vi "Actor Core.vi"(8 "error in":errorcluster, 11 "Panel Object Actions UI in":refnum<class "Panel Object Actions UI.lvclass">) -> (0 "error out":errorcluster, 3 "Actor out":refnum<class "Actor.lvclass">)   [LabVIEW 2019, in "Panel Object Actions UI.lvlib" / "Panel Object Actions UI.lvclass"]
doc: "The user interface for this panel.\n\n----\nPlease see the following web address for additional documentation and tutorial information:\nhttp://www.mooregoodideas.com/mgi-panel-manager/\n\nAuthor: Derek Trepanier\n\nCopyright (c) 2018, Moore Good Ideas, Inc.\n\nAll rights reserved.\n\nRedistribution and use in source and binary forms, with or without modification, are permitted provided that the following conditions are met:\n\n * Redistributions of source code must retain the above copyright notice, this list of conditions and the following disclaimer.\n * Redistributions in binary form must reproduce the above copyright notice, this list of conditions and the following disclaimer in the documentation and/or other materials provided with the distribution.\n * Neither the name of Moore Good Ideas, Inc. nor the names of its contributors may be used to endorse or promote products derived from this software without specific prior written permission.\n\nTHIS SOFTWARE IS PROVIDED BY THE COPYRIGHT HOLDERS AND CONTRIBUTORS \"AS IS\" AND ANY EXPRESS OR IMPLIED WARRANTIES, INCLUDING, BUT NOT LIMITED TO, THE IMPLIED WARRANTIES OF MERCHANTABILITY AND FITNESS FOR A PARTICULAR PURPOSE ARE DISCLAIMED. IN NO EVENT SHALL THE COPYRIGHT OWNER OR CONTRIBUTORS BE LIABLE FOR ANY DIRECT, INDIRECT, INCIDENTAL, SPECIAL, EXEMPLARY, OR CONSEQUENTIAL DAMAGES (INCLUDING, BUT NOT LIMITED TO, PROCUREMENT OF SUBSTITUTE GOODS OR SERVICES; LOSS OF USE, DATA, OR PROFITS; OR BUSINESS INTERRUPTION) HOWEVER CAUSED AND ON ANY THEORY OF LIABILITY, WHETHER IN CONTRACT, STRICT LIABILITY, OR TORT (INCLUDING NEGLIGENCE OR OTHERWISE) ARISING IN ANY WAY OUT OF THE USE OF THIS SOFTWARE, EVEN IF ADVISED OF THE POSSIBILITY OF SUCH DAMAGE."
uses:
  <resource>/dialog/QuickDrop/plugins/PaneRelief/Classes/Panel Object Actions UI/Panel Object Actions UI/Panel Object Actions UI.lvclass
  C:/Program Files (x86)/National Instruments/LabVIEW 2019/vi.lib/MGI/Panel Manager/Panel Actor/Panel Actor/Panel Actor.lvclass
  C:/Program Files (x86)/National Instruments/LabVIEW 2019/vi.lib/ActorFramework/Actor/Actor.lvclass
  <vilib>/ActorFramework/Actor/Actor.lvclass
  <resource>/dialog/QuickDrop/plugins/PaneRelief/Classes/Panel Object/Panel Object.lvclass
  <vilib>/ActorFramework/Actor/Actor.lvclass/Actor.ctl
  <resource>/dialog/QuickDrop/plugins/PaneRelief/Classes/Panel Object Actions UI/Panel Object Actions UI/Panel Object Actions UI.lvclass/Panel Object Actions UI.ctl
  <vilib>/ActorFramework/Message Enqueuer/Message Enqueuer.lvclass/Message Enqueuer.ctl
  <resource>/dialog/QuickDrop/plugins/PaneRelief/Typedefs/Scrollbar Visibility--Enum.ctl
  <resource>/dialog/QuickDrop/plugins/PaneRelief/Classes/Panel Object/Align Type--Enum.ctl
  <resource>/dialog/QuickDrop/plugins/PaneRelief/Classes/Panel Object/Distribution Type--Enum.ctl
  <vilib>/ActorFramework/Message Enqueuer/Enqueue.vi
  <resource>/dialog/QuickDrop/plugins/PaneRelief/Classes/Pane Relief Main UI/Pane Relief Main UI Messages/Panel Object Settings Changed Msg/Panel Object Settings Changed Msg.lvclass
  C:/Program Files (x86)/National Instruments/LabVIEW 2019/vi.lib/ActorFramework/Message/Message.lvclass
  <vilib>/ActorFramework/Message Priority Queue/Priority Enqueue.vi
  <vilib>/MGI/Panel Manager/Panel Actor/Panel Actor/Panel Actor.lvclass
  <vilib>/ActorFramework/Message Enqueuer/Message Enqueuer.lvclass
panel:
  in  "Scrollbars Off":bool
  in  "Scrollbars Off":bool
  in  "Unlock Splitters":bool
  in  "Lock Splitters":bool
  in  "Distribute Horizontally":bool
  in  "Distribute Vertically":bool
  in  "Set Color":bool
  in  "Scrollbars On":bool
  in  "Origin To (0,0)":bool
  in  "Align Right":bool
  in  "Align Bottom":bool
  in  "Align Left":bool
  in  "Align Top":bool
  in  "Color":u32(colorbox)
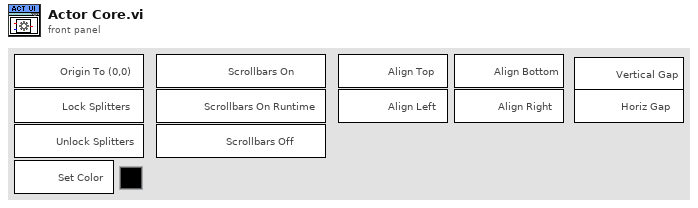
[diagram p1: front panel]
types:
  T1 = cluster{"Event Registration Refnum":refnum<event-registration>, "Pnl Actor":refnum<event-registration>}
  T2 = typedef "Scrollbar Visibility--Enum.ctl" = enum16{"On", "Off", "Off While Running"}
  T3 = typedef "Align Type--Enum.ctl" = enum16{"Top", "Bottom", "Left", "Right"}
  T4 = typedef "Distribution Type--Enum.ctl" = enum16{"Vertical", "Horizontal"}
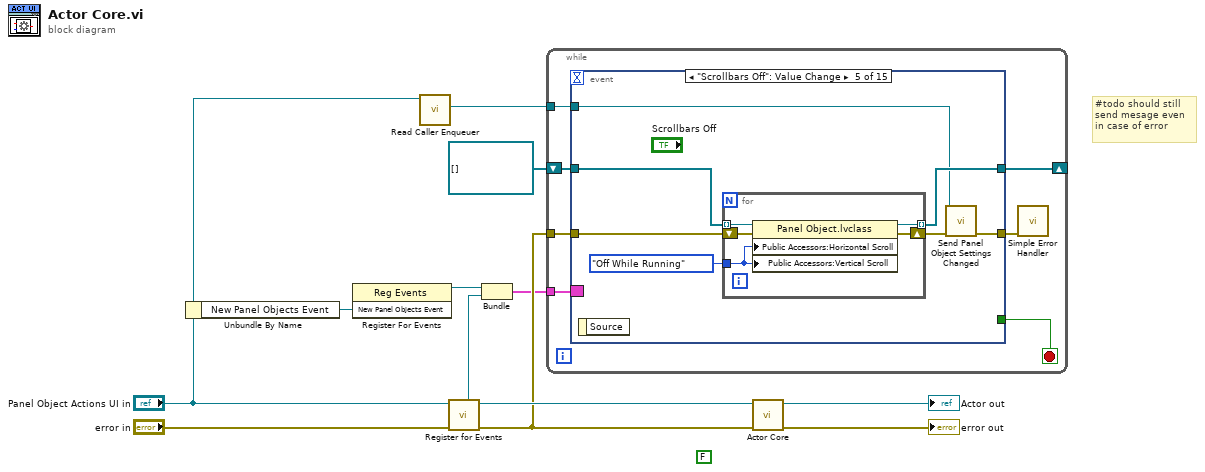
[diagram p0: block diagram]
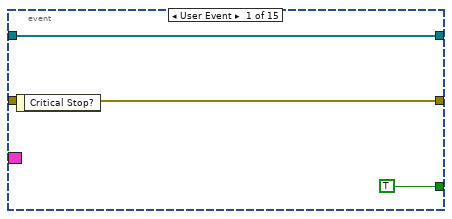
[diagram p2: hidden frame]
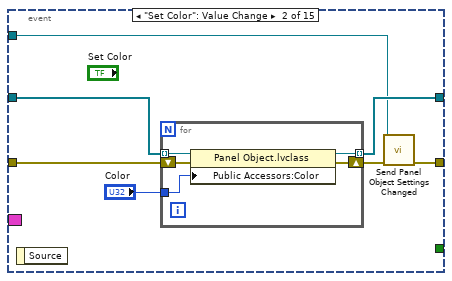
[diagram p3: hidden frame]
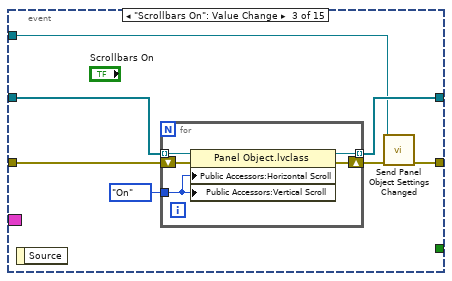
[diagram p4: hidden frame]
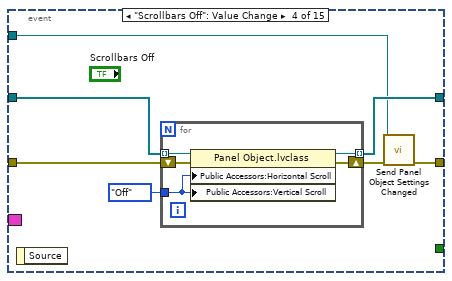
[diagram p5: hidden frame]
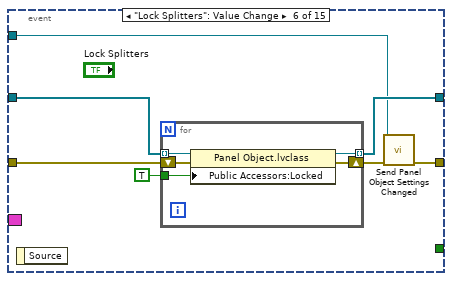
[diagram p6: hidden frame]
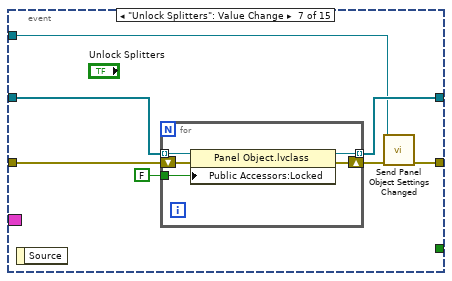
[diagram p7: hidden frame]
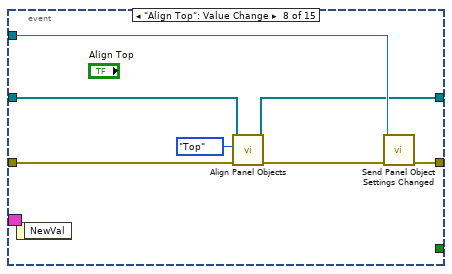
[diagram p8: hidden frame]
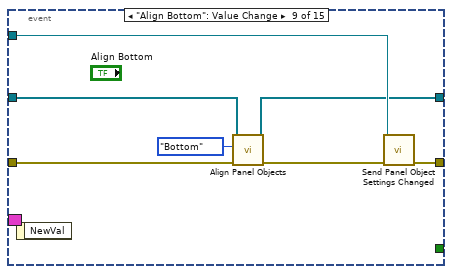
[diagram p9: hidden frame]
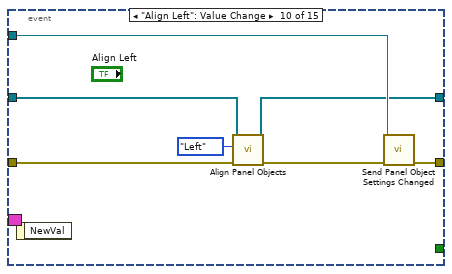
[diagram p10: hidden frame]
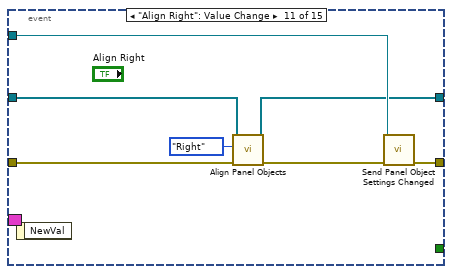
[diagram p11: hidden frame]
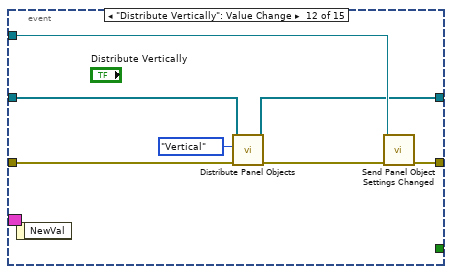
[diagram p12: hidden frame]
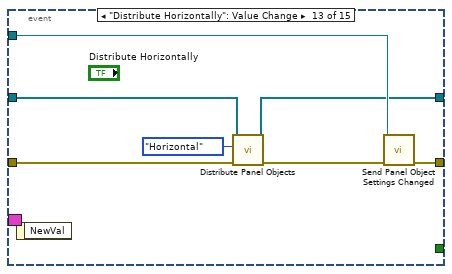
[diagram p13: hidden frame]
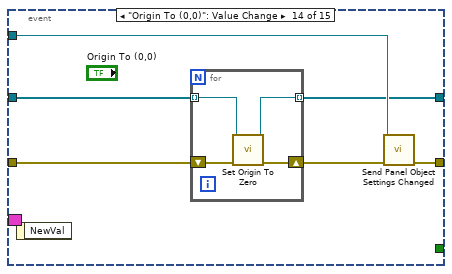
[diagram p14: hidden frame]
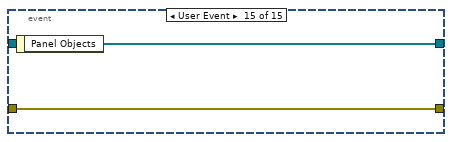
[diagram p15: hidden frame]
diagram:
  (unwired) FALSE
  # "#todo should still send mesage even in case of error"
  n1 = Unbundle By Name("Panel Object Actions UI in") -> ("New Panel Objects Event"=w6:refnum<user-event>)
  n2 = register-events(w6) -> (reference out=w10:refnum<event-registration>)  [unwired: 2 in, 1 out]
  n3 = call <vilib>:"Read Caller Enqueuer.vi"("Actor"="Panel Object Actions UI in") -> ("Caller Enqueuer"=w3:refnum<class "Message Enqueuer.lvclass">)  [unwired: 10 in]
  n4 = call <vilib>:"Register for Events.vi"("Error In"="error in", "Panel Actor in"="Panel Object Actions UI in") -> ("Error Out"=w5:errorcluster, "Panel Actor out"=w8:refnum<class "Panel Object Actions UI.lvclass">, "Pnl Actor"=w9:refnum<event-registration>)  [unwired: 6 in, 1 out]
  n5 = Bundle("Event Registration Refnum"=w10, "Pnl Actor"=w9) -> (w4:T1)  [unwired: 1 in]
  n6 = while {
    tunnel: w4 -> [w19]
    tunnel: w3 -> [w16]
    shift-right: [w15] -> _
    shift-left: refnum<class "Panel Object.lvclass">[] [] ("Panel Objects") -> [w14]
    tunnel: w5 -> [w17]
    stop <- w18 stop-if-true
    n7 = event shown="[4] \"Scrollbars Off\": Value Change" {
      selector: w19 -> [_ _ _ _ _ _ _ _ _ _ _ _ _ _ _]
      dyn-events: _ -> [_ _ _ _ _ _ _ _ _ _ _ _ _ _ _]
      timeout: _ -> [_ _ _ _ _ _ _ _ _ _ _ _ _ _ _]
      tunnel: [TRUE _ _ _ _ _ _ _ _ _ _ _ _ _ _] -> w18
      tunnel: w17 -> [w21 w26 w38 w50 w62 w74 w86 w99 w106 w113 w120 w127 w134 w140 w148]
      tunnel: [w21 w29 w41 w53 w65 w77 w89 w101 w108 w115 w122 w129 w136 w142 w148] -> w13
      tunnel: w16 -> [_ w24 w36 w48 w60 w72 w84 w100 w107 w114 w121 w128 w135 w141 _]
      tunnel: [w20 w25 w37 w49 w61 w73 w85 w96 w103 w110 w117 w124 w131 w137 w147] -> w15
      tunnel: w14 -> [w20 w28 w40 w52 w64 w76 w88 w97 w104 w111 w118 w125 w132 w138 _]
      event User Event {
        n8 = event-data() -> ()  [unwired: 1 in, 1 out]
      }
      event "Set Color": Value Change {
        n9 = event-data() -> ()  [unwired: 1 in, 1 out]
        n10 = for {
          tunnel: w28 -> [w34] mode=indexing
          shift-right: [w33] -> w27
          shift-left: w26 -> [w32]
          tunnel: [w31] -> w25 mode=indexing
          tunnel: "Color" -> [w30]
          n11 = property class="Panel Object.lvclass"(reference=w34, error in=w32, "Public Accessors:Color"=w30) -> (reference out=w31:refnum<class "Panel Object.lvclass">, error out=w33:errorcluster)
        }
        n12 = call <resource>:"Send Panel Object Settings Changed.vi"("error in (no error)"=w27, "Message Enqueuer"=w24) -> ("error out"=w29:errorcluster)  [unwired: 8 in, 1 out]
      }
      event "Scrollbars On": Value Change {
        n13 = event-data() -> ()  [unwired: 1 in, 1 out]
        n14 = for {
          tunnel: w40 -> [w46] mode=indexing
          shift-right: [w45] -> w39
          shift-left: w38 -> [w44]
          tunnel: [w43] -> w37 mode=indexing
          tunnel: Scrollbar_Visibility--Enum."On" ("Vertical Scroll") -> [w42]
          n15 = property class="Panel Object.lvclass"(reference=w46, error in=w44, "Public Accessors:Horizontal Scroll"=w42, "Public Accessors:Vertical Scroll"=w42) -> (reference out=w43:refnum<class "Panel Object.lvclass">, error out=w45:errorcluster)
        }
        n16 = call <resource>:"Send Panel Object Settings Changed.vi"("error in (no error)"=w39, "Message Enqueuer"=w36) -> ("error out"=w41:errorcluster)  [unwired: 8 in, 1 out]
      }
      event "Scrollbars Off": Value Change {
        n17 = event-data() -> ()  [unwired: 1 in, 1 out]
        n18 = for {
          tunnel: w52 -> [w58] mode=indexing
          shift-right: [w57] -> w51
          shift-left: w50 -> [w56]
          tunnel: [w55] -> w49 mode=indexing
          tunnel: Scrollbar_Visibility--Enum."Off" ("Vertical Scroll") -> [w54]
          n19 = property class="Panel Object.lvclass"(reference=w58, error in=w56, "Public Accessors:Horizontal Scroll"=w54, "Public Accessors:Vertical Scroll"=w54) -> (reference out=w55:refnum<class "Panel Object.lvclass">, error out=w57:errorcluster)
        }
        n20 = call <resource>:"Send Panel Object Settings Changed.vi"("error in (no error)"=w51, "Message Enqueuer"=w48) -> ("error out"=w53:errorcluster)  [unwired: 8 in, 1 out]
      }
      event "Scrollbars Off": Value Change {
        n21 = event-data() -> ()  [unwired: 1 in, 1 out]
        n22 = for {
          tunnel: w64 -> [w70] mode=indexing
          shift-right: [w69] -> w63
          shift-left: w62 -> [w68]
          tunnel: [w67] -> w61 mode=indexing
          tunnel: Scrollbar_Visibility--Enum."Off While Running" ("Vertical Scroll") -> [w66]
          n23 = property class="Panel Object.lvclass"(reference=w70, error in=w68, "Public Accessors:Horizontal Scroll"=w66, "Public Accessors:Vertical Scroll"=w66) -> (reference out=w67:refnum<class "Panel Object.lvclass">, error out=w69:errorcluster)
        }
        n24 = call <resource>:"Send Panel Object Settings Changed.vi"("error in (no error)"=w63, "Message Enqueuer"=w60) -> ("error out"=w65:errorcluster)  [unwired: 8 in, 1 out]
      }
      event "Lock Splitters": Value Change {
        n25 = event-data() -> ()  [unwired: 1 in, 1 out]
        n26 = for {
          tunnel: w76 -> [w82] mode=indexing
          shift-right: [w81] -> w75
          shift-left: w74 -> [w80]
          tunnel: [w79] -> w73 mode=indexing
          tunnel: TRUE -> [w78]
          n27 = property class="Panel Object.lvclass"(reference=w82, error in=w80, "Public Accessors:Locked"=w78) -> (reference out=w79:refnum<class "Panel Object.lvclass">, error out=w81:errorcluster)
        }
        n28 = call <resource>:"Send Panel Object Settings Changed.vi"("error in (no error)"=w75, "Message Enqueuer"=w72) -> ("error out"=w77:errorcluster)  [unwired: 8 in, 1 out]
      }
      event "Unlock Splitters": Value Change {
        n29 = event-data() -> ()  [unwired: 1 in, 1 out]
        n30 = for {
          tunnel: w88 -> [w94] mode=indexing
          shift-right: [w93] -> w87
          shift-left: w86 -> [w92]
          tunnel: [w91] -> w85 mode=indexing
          tunnel: FALSE -> [w90]
          n31 = property class="Panel Object.lvclass"(reference=w94, error in=w92, "Public Accessors:Locked"=w90) -> (reference out=w91:refnum<class "Panel Object.lvclass">, error out=w93:errorcluster)
        }
        n32 = call <resource>:"Send Panel Object Settings Changed.vi"("error in (no error)"=w87, "Message Enqueuer"=w84) -> ("error out"=w89:errorcluster)  [unwired: 8 in, 1 out]
      }
      event "Align Top": Value Change {
        n33 = event-data() -> ()  [unwired: 1 in, 1 out]
        n34 = call <resource>:"Align Panel Objects.vi"("error in (no error)"=w99, "Align Type"=Align_Type--Enum."Top", "Panel Objects in"=w97) -> ("error out"=w98:errorcluster, "Panel Objects out"=w96:refnum<class "Panel Object.lvclass">[])  [unwired: 7 in]
        n35 = call <resource>:"Send Panel Object Settings Changed.vi"("error in (no error)"=w98, "Message Enqueuer"=w100) -> ("error out"=w101:errorcluster)  [unwired: 8 in, 1 out]
      }
      event "Align Bottom": Value Change {
        n36 = event-data() -> ()  [unwired: 1 in, 1 out]
        n37 = call <resource>:"Align Panel Objects.vi"("error in (no error)"=w106, "Align Type"=Align_Type--Enum."Bottom", "Panel Objects in"=w104) -> ("error out"=w105:errorcluster, "Panel Objects out"=w103:refnum<class "Panel Object.lvclass">[])  [unwired: 7 in]
        n38 = call <resource>:"Send Panel Object Settings Changed.vi"("error in (no error)"=w105, "Message Enqueuer"=w107) -> ("error out"=w108:errorcluster)  [unwired: 8 in, 1 out]
      }
      event "Align Left": Value Change {
        n39 = event-data() -> ()  [unwired: 1 in, 1 out]
        n40 = call <resource>:"Align Panel Objects.vi"("error in (no error)"=w113, "Align Type"=Align_Type--Enum."Left", "Panel Objects in"=w111) -> ("error out"=w112:errorcluster, "Panel Objects out"=w110:refnum<class "Panel Object.lvclass">[])  [unwired: 7 in]
        n41 = call <resource>:"Send Panel Object Settings Changed.vi"("error in (no error)"=w112, "Message Enqueuer"=w114) -> ("error out"=w115:errorcluster)  [unwired: 8 in, 1 out]
      }
      event "Align Right": Value Change {
        n42 = event-data() -> ()  [unwired: 1 in, 1 out]
        n43 = call <resource>:"Align Panel Objects.vi"("error in (no error)"=w120, "Align Type"=Align_Type--Enum."Right", "Panel Objects in"=w118) -> ("error out"=w119:errorcluster, "Panel Objects out"=w117:refnum<class "Panel Object.lvclass">[])  [unwired: 7 in]
        n44 = call <resource>:"Send Panel Object Settings Changed.vi"("error in (no error)"=w119, "Message Enqueuer"=w121) -> ("error out"=w122:errorcluster)  [unwired: 8 in, 1 out]
      }
      event "Distribute Vertically": Value Change {
        n45 = event-data() -> ()  [unwired: 1 in, 1 out]
        n46 = call <resource>:"Distribute Panel Objects.vi"("error in (no error)"=w127, "Distribution Type"=Distribution_Type--Enum."Vertical", "Panel Objects in"=w125) -> ("error out"=w126:errorcluster, "Panel Objects out"=w124:refnum<class "Panel Object.lvclass">[])  [unwired: 7 in]
        n47 = call <resource>:"Send Panel Object Settings Changed.vi"("error in (no error)"=w126, "Message Enqueuer"=w128) -> ("error out"=w129:errorcluster)  [unwired: 8 in, 1 out]
      }
      event "Distribute Horizontally": Value Change {
        n48 = event-data() -> ()  [unwired: 1 in, 1 out]
        n49 = call <resource>:"Distribute Panel Objects.vi"("error in (no error)"=w134, "Distribution Type"=Distribution_Type--Enum."Horizontal", "Panel Objects in"=w132) -> ("error out"=w133:errorcluster, "Panel Objects out"=w131:refnum<class "Panel Object.lvclass">[])  [unwired: 7 in]
        n50 = call <resource>:"Send Panel Object Settings Changed.vi"("error in (no error)"=w133, "Message Enqueuer"=w135) -> ("error out"=w136:errorcluster)  [unwired: 8 in, 1 out]
      }
      event "Origin To (0,0)": Value Change {
        n51 = event-data() -> ()  [unwired: 1 in, 1 out]
        n52 = for {
          tunnel: w138 -> [w144] mode=indexing
          tunnel: [w143] -> w137 mode=indexing
          shift-right: [w145] -> w139
          shift-left: w140 -> [w146]
          n53 = call-dynamic "Set Origin To Zero.vi"("error in (no error)"=w146, "Panel Object in"=w144) -> ("error out"=w145:errorcluster, "Panel Object out"=w143:refnum<class "Panel Object.lvclass">)  [unwired: 8 in]
        }
        n54 = call <resource>:"Send Panel Object Settings Changed.vi"("error in (no error)"=w139, "Message Enqueuer"=w141) -> ("error out"=w142:errorcluster)  [unwired: 8 in, 1 out]
      }
      event User Event {
        n55 = event-data() -> ("Panel Objects"=w147:refnum<class "Panel Object.lvclass">[])  [unwired: 1 in]
      }
    }
    n56 = call <vilib>:"Simple Error Handler.vi"("error in (no error)"=w13) -> ()  [unwired: 4 in, 5 out]
  }
  n57 = call-parent "Actor Core.vi"("error in"=w5, "Panel Actor in"=w8) -> ("error out"=→"error out":errorcluster, "Actor out"=→"Actor out":refnum<class "Actor.lvclass">)  [unwired: 8 in]
